vi "Test Recursive Tree View.vi"() -> ()   [LabVIEW 2020]
panel:
  in  "Depth":i32=3
  in  "Indent":i32
  in  "Tree":string(tree)
  in  "Path":path=path "C:/Users/gsfcprime/Documents/LabVIEW Data/PRIME FITS Images"
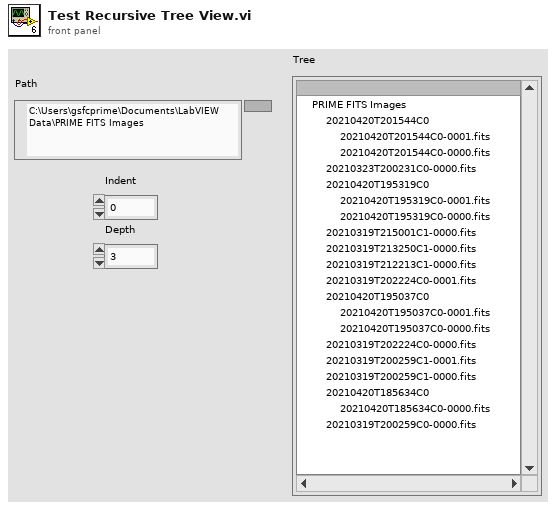
[diagram p1: front panel]
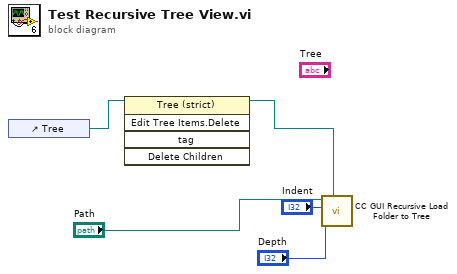
[diagram p0: block diagram]
diagram:
  n1 = control-ref of="Tree"() -> (w2:refnum<vi>)
  n2 = invoke on="Invoke Node" class="Tree (strict)" method="Edit Tree Items.Delete"(reference=w2) -> (reference out=w1:refnum<vi>)  [unwired: 4 in, 4 out]
  n3 = call "CC GUI Recursive Load Folder to Tree.vi"("Tree Ref"=w1, "Depth"="Depth", "Indent"="Indent", "Path"="Path") -> ()  [unwired: 7 in, 1 out]
